vi "update_pipette_counter.vi"(8 "error in (no error)":errorcluster, 11 "PrepLineObject in":refnum<class "PrepLineObject.lvclass">) -> (0 "error out":errorcluster, 3 "PrepLineObject out":refnum<class "PrepLineObject.lvclass">)   [LabVIEW 2017]
doc: "checks whether or not the switch is a switch of a pipette (inner-switch).\nIf so the VI updates the piptte counter in the PipObject AND also updates the counter in the Pipettes.ini file"
uses:
  Classes/PrepLineObject/PrepLineObject.lvclass
  <vilib>/Utility/config.llb/Write Key (Double).vi
  Classes/Pipette/Pipette.lvclass
  <vilib>/Utility/config.llb/NI_LVConfig.lvlib
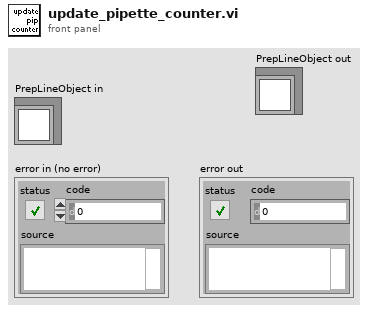
[diagram p1: front panel]
types:
  T1 = typedef "NI_LVConfig.lvlib/Config Data RefNum.ctl" = refnum<k1>
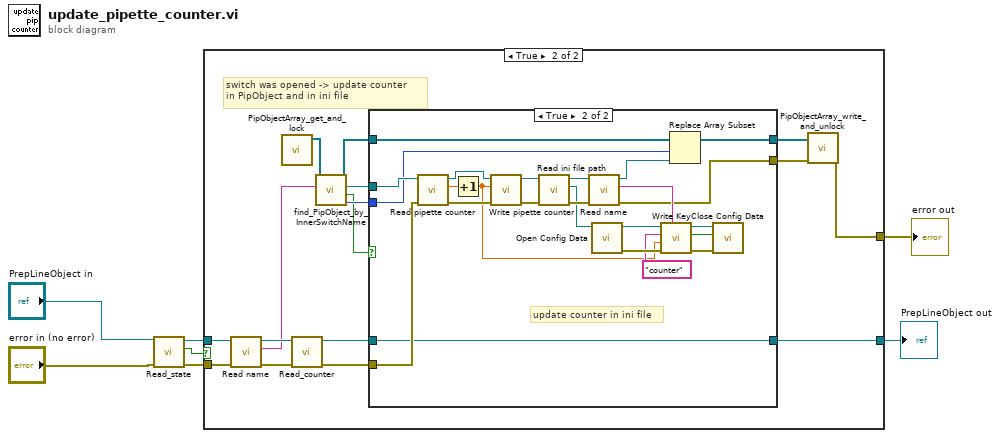
[diagram p0: block diagram]
diagram:
  n1 = call-dynamic "Read_state.vi"("error in (no error)"="error in (no error)", "PrepLineObject in"="PrepLineObject in") -> ("error out"=w6:errorcluster, "state"=w4:bool, "PrepLineObject out"=w5:refnum<class "PrepLineObject.lvclass">)  [unwired: 7 in]
  n2 = case shown="True" w4 {
    tunnel: [w9 w13] -> w7
    tunnel: w6 -> [w9 w23]
    tunnel: w5 -> [w8 w24]
    tunnel: [w8 w10] -> w1
    frame False {
      # "don't update"
    }
    frame True {
      # "switch was opened -> update counter\nin PipObject and in ini file"
      n3 = call-dynamic "Read name.vi"("error in (no error)"=w23, "PrepLineObject in"=w24) -> ("error out"=w21:errorcluster, "name"=w20:string, "PrepLineObject out"=w22:refnum<class "PrepLineObject.lvclass">)  [unwired: 7 in]
      n4 = call "PipObjectArray_get_and_lock.vi"() -> ("PipObjects"=w25:refnum<class "Pipette.lvclass">[])  [unwired: 10 in, 1 out]
      n5 = call-dynamic "Read_counter.vi"("error in (no error)"=w21, "PrepLineObject in"=w22) -> ("error out"=w18:errorcluster, "PrepLineObject out"=w11:refnum<class "PrepLineObject.lvclass">)  [unwired: 7 in, 1 out]
      n6 = call "find_PipObject_by_InnerSwitchName.vi"("inner switch name"=w20, "PipObj Array in"=w25) -> ("index of Object in Array"=w16:i32, "found?"=w12:bool, "found PipObj out"=w19:refnum<class "Pipette.lvclass">, "PipObj Array out"=w17:refnum<class "Pipette.lvclass">[])  [unwired: 6 in]
      n7 = case shown="True" w12 {
        tunnel: w19 -> [_ w52]
        tunnel: w18 -> [w27 w48]
        tunnel: w17 -> [w28 w39]
        tunnel: w16 -> [_ w38]
        tunnel: [w28 w36] -> w15
        tunnel: [w27 w30] -> w14
        tunnel: w11 -> [w26 w29]
        tunnel: [w26 w29] -> w10
        frame False {
          # "it's not a pipette"
        }
        frame True {
          # "update counter in ini file"
          n8 = call-dynamic "Read pipette counter.vi"("error in (no error)"=w48, "Pipette in"=w52) -> ("error out"=w49:errorcluster, "pipette counter"=w51:dbl, "Pipette out"=w50:refnum<class "Pipette.lvclass">)  [unwired: 7 in]
          n9 = Increment(x=w51) -> (x+1=w40:dbl)
          n10 = call-dynamic "Write pipette counter.vi"("error in (no error)"=w49, "pipette counter"=w40, "Pipette in"=w50) -> ("error out"=w33:errorcluster, "Pipette out"=w35:refnum<class "Pipette.lvclass">)  [unwired: 7 in]
          n11 = call-dynamic "Read ini file path.vi"("error in (no error)"=w33, "Pipette in"=w35) -> ("error out"=w32:errorcluster, "ini file path"=w31:path, "Pipette out"=w34:refnum<class "Pipette.lvclass">)  [unwired: 7 in]
          n12 = call-dynamic "Read name.vi"("error in (no error)"=w32, "Pipette in"=w34) -> ("error out"=w30:errorcluster, "name"=w41:string, "Pipette out"=w37:refnum<class "Pipette.lvclass">)  [unwired: 7 in]
          n13 = call <vilib>:"Open Config Data.vi"("configuration file path"=w31) -> ("error out"=w47:errorcluster, "refnum"=w46:T1)  [unwired: 8 in, 1 out]
          n14 = call-poly <vilib>:"Write Key.vi"("section"=w41, "error in (no error)"=w47, "value"=w40, "key"="counter", "refnum"=w46) -> ("error out"=w44:errorcluster, "found?"=w43:bool, "refnum out"=w42:T1)  [unwired: 4 in]
          n15 = Replace Array Subset(array=w39, new element=w37, index=w38) -> (w36:refnum<class "Pipette.lvclass">[])
          n16 = call <vilib>:"Close Config Data.vi"("error in (no error)"=w44, "write file if changed (T)"=w43, "refnum"=w42) -> ()  [unwired: 7 in, 2 out]
        }
      }
      n17 = call "PipObjectArray_write_and_unlock.vi"("error in (no error)"=w14, "PipObjects"=w15) -> ("error out"=w13:errorcluster)  [unwired: 9 in]
    }
  }
  "error out" <- w7
  "PrepLineObject out" <- w1
